vi "Get Named Elements.vi"(10 "names":string[](array[string]), 11 "tokens":cluster{"token type":T2, T3}[](array[cluster])) -> (3 "Found Token Info":T1(array[cluster]))   [LabVIEW 2020, in "Multi Error Cluster.lvlib"]
doc: "Search the root level of the tokenized JSON identifying fields with the names of interest. Outputs contain strings, but are not necessarily in the requested order."
uses:
  <vilib>/MultiError/TokenizeJSON/Multi Error Cluster.lvlib
  <vilib>/MultiError/TokenizeJSON/JSON Token Values.ctl
  <vilib>/MultiError/Errors Cluster Multiple Errors/JSON Token Descriptor.ctl
  <vilib>/MultiError/TokenizeJSON/JSON Raw Token Values.ctl
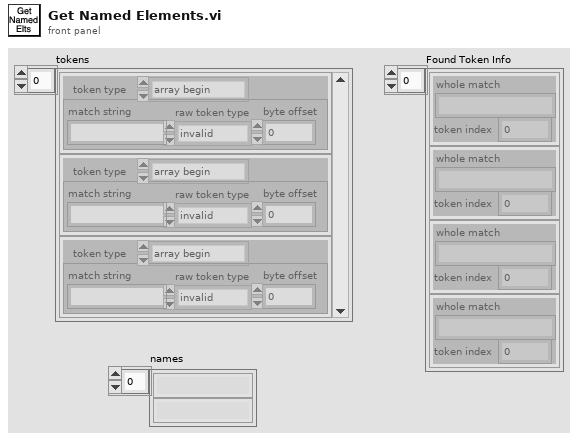
[diagram p1: front panel]
types:
  T1 = cluster{"whole match":string, "token index":i32}[]
  T2 = typedef "Multi Error Cluster.lvlib/JSON Token Values.ctl" = enum32{"array begin", "array end", "object begin", "object end", "value", "invalid", "name"}
  T3 = typedef "Multi Error Cluster.lvlib/JSON Token Descriptor.ctl" = cluster{"match string":string, "raw token type":T4, "byte offset ":i32}
  T4 = typedef "Multi Error Cluster.lvlib/JSON Raw Token Values.ctl" = enum32{"{", "}", "[", "]", ",", ":", "\"", "number", "string", "true", "false", "null", "invalid"}
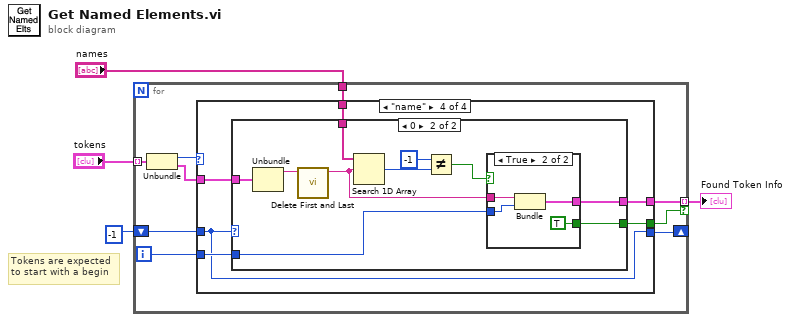
[diagram p0: block diagram]
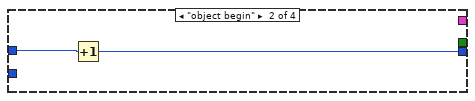
[diagram p3: hidden frame]
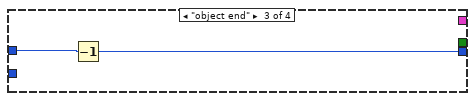
[diagram p4: hidden frame]
diagram:
  # "Tokens are expected\nto start with a begin"
  n1 = for {
    tunnel: "tokens" -> [w13] mode=indexing
    tunnel: "names" -> [w12]
    tunnel: [w10] -> w3 mode=indexing if=w9
    shift-right: [w7] -> _
    shift-left: -1 -> [w8]
    i -> [w11]
    n2 = Unbundle(w13) -> ("token type"=w6:T2, w5:T3)
    n3 = case shown="\"name\"" w6 {
      tunnel: w5 -> [_ _ _ w24]
      tunnel: w12 -> [_ _ _ w23]
      tunnel: w11 -> [_ _ _ w22]
      tunnel: [_ _ _ w21] -> w10
      tunnel: [_ _ _ w20] -> w9
      tunnel: w8 -> [w14 w16 w18 w19]
      tunnel: [w14 w15 w17 w19] -> w7
      frame Default {
      }
      frame "object begin" {
        n4 = Increment(x=w16) -> (x+1=w15:i32)
      }
      frame "object end" {
        n5 = Decrement(x=w18) -> (x-1=w17:i32)
      }
      frame "name" {
        n6 = case shown="0" w19 {
          tunnel: w24 -> [_ w34]
          tunnel: w23 -> [_ w33]
          tunnel: w22 -> [_ w29]
          tunnel: [_ w28] -> w21
          tunnel: [_ w27] -> w20
          frame Default {
          }
          frame 0 {
            n7 = Unbundle(w34) -> ("match string"=w26:string)  [unwired: 2 out]
            n8 = call <vilib>:"Delete First and Last.vi"("string in"=w26) -> ("string subset"=w25:string)  [unwired: 10 in]
            n9 = Search 1D Array(1D array=w33, element=w25) -> (index of element=w32:i32)  [unwired: 1 in]
            n10 = Not Equal?(x=-1, y=w32) -> (x != y?=w30:bool)
            n11 = case shown="True" w30 {
              tunnel: w25 -> [_ w38]
              tunnel: w29 -> [_ w35]
              tunnel: [_ w37] -> w28
              tunnel: [_ TRUE] -> w27
              frame False {
              }
              frame True {
                n12 = Bundle("string subset"=w38, w35) -> (w37:cluster{"string subset":string, i32})  [unwired: 1 in]
              }
            }
          }
        }
      }
    }
  }
  "Found Token Info" <- w3
